vi "RotStageParams.vi"(0 "Rot lines per plane":T1(ring)=enum."400", 1 "Sector Angle":i32(slide)=360 min=0 max=360 step=45 scale=0.0..360.0) -> (2 "Valid combo":bool, 3 "Number of scan lines":i32, 4 "distance between scans":i32)   [LabVIEW 2022 SP3]
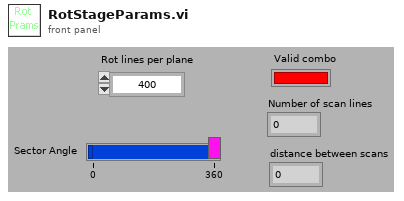
[diagram p1: front panel]
types:
  T1 = enum16{"50", "100", "200", "250", "400", "500", "1000"}
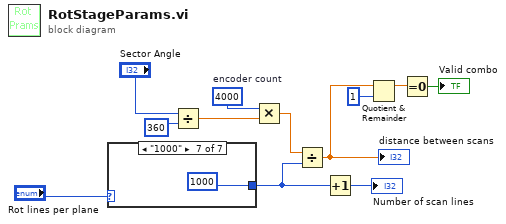
[diagram p0: block diagram]
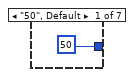
[diagram p2: hidden frame]
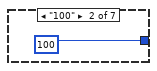
[diagram p3: hidden frame]
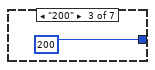
[diagram p4: hidden frame]
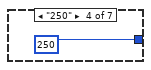
[diagram p5: hidden frame]
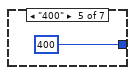
[diagram p6: hidden frame]
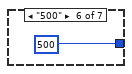
[diagram p7: hidden frame]
diagram:
  w7 = 4000  # encoder count
  n1 = case shown="\"1000\"" "Rot lines per plane" {
    tunnel: [50 100 200 250 400 500 1000] -> w10
    frame "50", Default {
    }
    frame "100" {
    }
    frame "200" {
    }
    frame "250" {
    }
    frame "400" {
    }
    frame "500" {
    }
    frame "1000" {
    }
  }
  n2 = Divide(x="Sector Angle", y=360) -> (x/y=w8:dbl)
  n3 = Multiply(x=w7, y=w8) -> (x*y=w6:dbl)
  n4 = Divide(x=w6, y=w10) -> (x/y=w2:dbl)
  "distance between scans" <- w2
  n5 = Increment(x=w10) -> (x+1=→"Number of scan lines":i32)
  n6 = Quotient & Remainder(x=w2, y=1) -> (x-y*floor(x/y)=w4:dbl)  [unwired: 1 out]
  n7 = Equal To 0?(x=w4) -> (x = 0?=→"Valid combo":bool)
